vi "OpenBlockDiagram.vi"(8 "ErrorIn":errorcluster, 11 "ObjectIn":refnum<class "FrontPanelControl.lvclass">) -> (0 "ErrorOut":errorcluster, 3 "ObjectOut":refnum<class "FrontPanelControl.lvclass">)   [LabVIEW 2021, in "FrontPanelControl.lvclass"]
uses:
  FrontPanelControl.lvclass
  FrontPanelControl.lvclass/FrontPanelControl.ctl
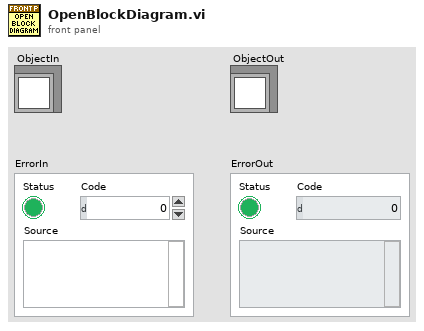
[diagram p1: front panel]
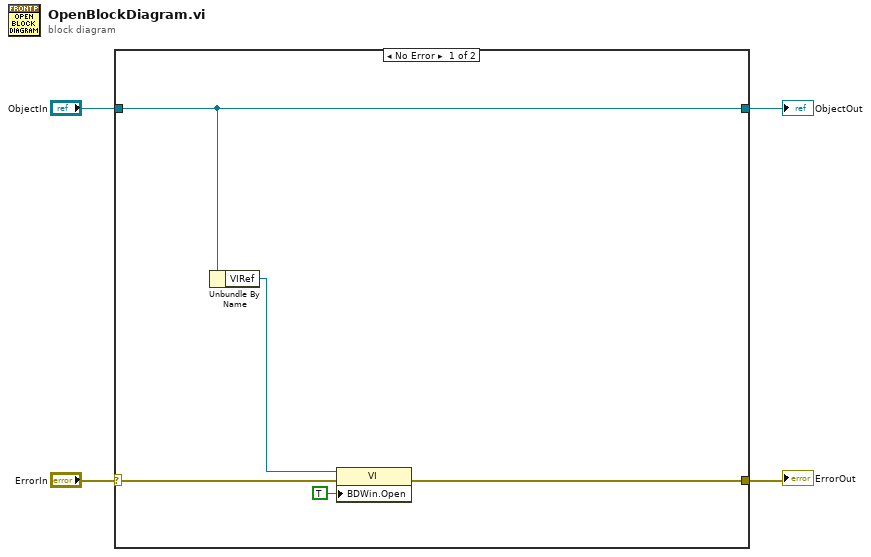
[diagram p0: block diagram]
diagram:
  n1 = case shown="No Error" "ErrorIn" {
    selector: "ErrorIn" -> [w9 w11]
    tunnel: [w8 w11] -> w3
    tunnel: [w7 w10] -> w1
    tunnel: "ObjectIn" -> [w7 w10]
    frame No Error {
      n2 = Unbundle By Name(w7) -> ("VIRef"=w6:refnum<vi>)
      n3 = property class="VI"(reference=w6, error in=w9, "BDWin.Open"=TRUE ("Block Diagram Window:Open")) -> (error out=w8:errorcluster)  [unwired: 1 out]
    }
    frame Error {
    }
  }
  "ErrorOut" <- w3
  "ObjectOut" <- w1
